vi "Xml_Save_Excit_Table.vi"(8 "error in (no error)":errorcluster, 11 "Refnum Clust":refnum<vi>) -> (0 "error out":errorcluster, 3 "XML String Out":string)   [LabVIEW 2017]
uses:
  controls/EXCIT_Table.ctl
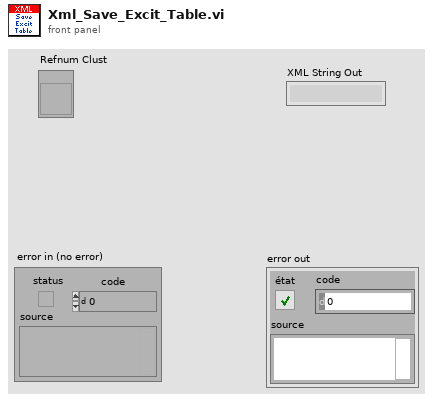
[diagram p1: front panel]
types:
  T1 = typedef "EXCIT_Table.ctl" = cluster{"Number of Excits":u16, "Number of Ejects":u16, "Sampling Frequency":dbl, "Waveforms Table":string[][]}
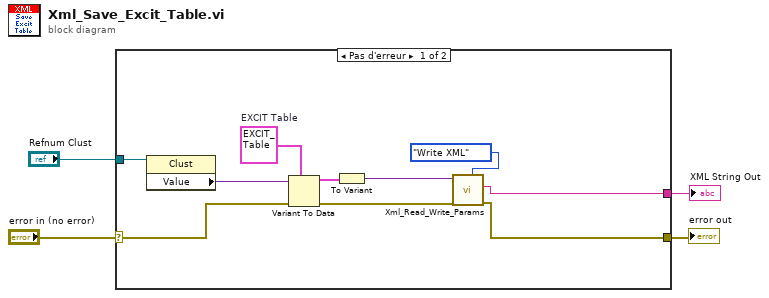
[diagram p0: block diagram]
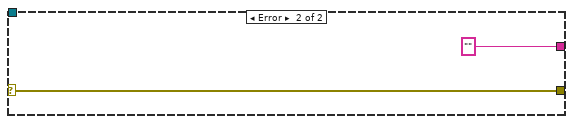
[diagram p2: hidden frame]
diagram:
  n1 = case shown="Pas d'erreur" "error in (no error)" {
    selector: "error in (no error)" -> [w14 w16]
    tunnel: [w13 w16] -> w3
    tunnel: [w12 "" ("XML String Out")] -> w2
    tunnel: "Refnum Clust" -> [w7 _]
    frame No Error {
      w5 = T1 {"Number of Excits"=0, "Number of Ejects"=0, "Sampling Frequency"=0.0, "Waveforms Table"=[["Excit1", "name", "Swift", "0.5", "1200", "70", "150", "550", "0", "0", "0"]]}  # EXCIT Table
      n2 = property class="Clust"(reference=w7) -> ("Value"=w8:variant)  [unwired: 1 in, 2 out]
      n3 = Variant To Data(error in=w14, type=w5, Variant=w8) -> (data=w6:T1, error out=w9:errorcluster)
      n4 = To Variant(anything=w6) -> (Variant=w11:variant)
      n5 = call "Xml_Read_Write_Params.vi"("Variant"=w11, "error in (no error)"=w9, "Command"=enum16{"Read XML", "Set", "Get", "Write XML"}."Write XML") -> ("XML String Out"=w12:string, "error out"=w13:errorcluster)  [unwired: 4 in, 1 out]
    }
    frame Error {
    }
  }
  "error out" <- w3
  "XML String Out" <- w2
